vi "trova_armoniche.vi"(5 "Waveform":waveform(dbl)) -> ()   [LabVIEW 2012]
uses:
  <vilib>/measure/NI_MAPro.lvlib
  <vilib>/measure/maspectr.llb/FFT Spectrum (Mag-Phase) for 1 Chan.vi
  <vilib>/Analysis/4window.llb/windowTd.ctl
  <vilib>/Analysis/NI_AALPro.lvlib
panel:
  out "armoniche":T1(array[cluster])
  in  "armonica":cluster{"nArmonica":i32, "freq":dbl, "Vrms":dbl}={"nArmonica"=1, "freq"=0.0, "Vrms"=0.0} {"Vrms" min=0.0; "nArmonica" min=1 step=1; "freq" min=0.0}
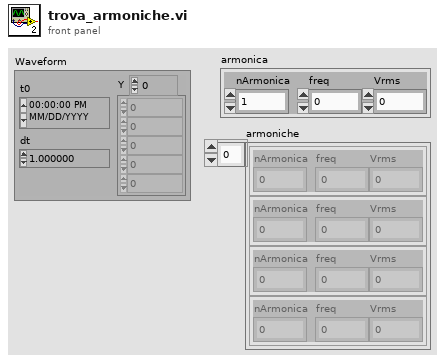
[diagram p1: front panel]
types:
  T1 = cluster{"nArmonica":i32, "freq":dbl, "Vrms":dbl}[]
  T2 = typedef "NI_AALPro.lvlib/windowTd.ctl" = u32
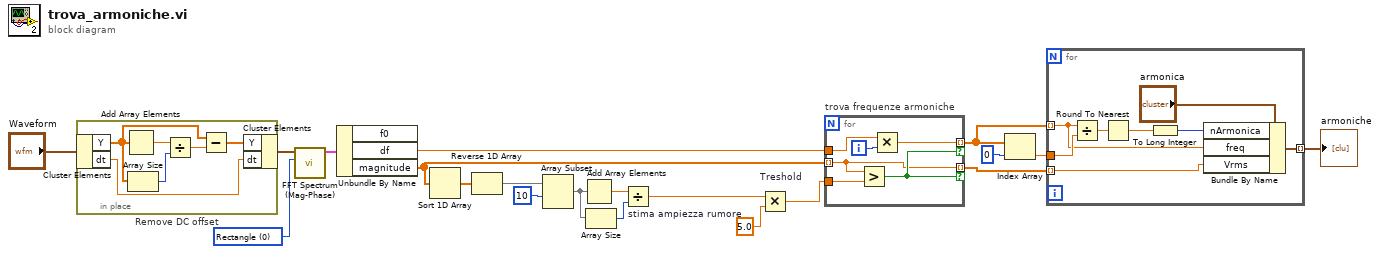
[diagram p0: block diagram]
diagram:
  w6 = T2 0 items=["Rectangle"=0, "Hanning"=1, "Hamming"=2, "Blackman-Harris"=3, "Exact Blackman"=4, "Blackman"=5, "Flat Top"=6, "4 Term B-Harris "=7, "7 Term B-Harris"=8, "Low Sidelobe"=9, "Blackman Nuttall"=11, "Triangle"=30, "Bartlett-Hanning"=31, "Bohman"=32, "Parzen"=33, "Welch"=34, "Kaiser"=60, "Dolph-Chebyshev"=61, "Gaussian"=62] ("window")
  n1 = in-place "Remove DC offset" {
    n2 = in-place-cluster #1("Waveform") -> ("Y"=w23:dbl[], "dt"=w26:dbl)
    n3 = Add Array Elements(numeric array=w23) -> (sum=w25:dbl)
    n4 = Array Size(array=w23) -> (size(s)=w24:i32)
    n5 = Divide(x=w25, y=w24) -> (x/y=w22:dbl)
    n6 = Subtract(x=w23, y=w22) -> (x-y=w21:dbl[])
    n7 = in-place-cluster #1("Y"=w21, "dt"=w26) -> (w16:waveform(dbl))
  }
  n8 = call-poly <vilib>:"FFT Spectrum (Mag-Phase).vi"("window"=w6, "time signal"=w16) -> ("magnitude"=w20:cluster{"f0":dbl, "df":dbl, "magnitude":dbl[]})  [unwired: 5 in, 4 out]
  n9 = Unbundle By Name(w20) -> ("df"=w17:dbl, "magnitude"=w13:dbl[])  [unwired: 1 out]
  n10 = Sort 1D Array(array=w13) -> (sorted array=w9:dbl[])
  n11 = Reverse 1D Array(array=w9) -> (reversed array=w10:dbl[])
  n12 = Array Subset(array=w10, index=10) -> (w18:dbl[])  [unwired: 1 in]
  n13 = Add Array Elements(numeric array=w18) -> (sum=w7:dbl)
  n14 = Array Size(array=w18) -> (size(s)=w8:i32)
  n15 = Divide "stima ampiezza rumore"(x=w7, y=w8) -> (x/y=w11:dbl)
  n16 = Multiply "Treshold"(x=w11, y=5.0) -> (x*y=w14:dbl)
  n17 = for "trova frequenze armoniche" {
    tunnel: w13 -> [w27] mode=indexing
    tunnel: w14 -> [w32]
    tunnel: w17 -> [w29]
    tunnel: [w30] -> w3 mode=indexing if=w28
    tunnel: [w27] -> w2 mode=indexing if=w28
    i -> [w31]
    n18 = Greater?(x=w27, y=w32) -> (0:w28:bool)
    n19 = Multiply(x=w29, y=w31) -> (x*y=w30:dbl)
  }
  n20 = Index Array(array=w3, index=0) -> (element=w4:dbl)
  n21 = for {
    tunnel: w3 -> [w34] mode=indexing
    tunnel: w4 -> [w40]
    tunnel: w2 -> [w33] mode=indexing
    tunnel: [w36] -> w1 mode=indexing
    n22 = Divide(x=w34, y=w40) -> (x/y=w39:dbl)
    n23 = Round To Nearest(number=w39) -> (nearest integer value=w38:dbl)
    n24 = To Long Integer(number=w38) -> (32bit integer=w35:i32)
    n25 = Bundle By Name(cluster="armonica", "nArmonica"=w35, "freq"=w34, "Vrms"=w33) -> (w36:cluster{"nArmonica":i32, "freq":dbl, "Vrms":dbl})
  }
  "armoniche" <- w1
